vi "Get VIPM Package Installed Filepaths.vi"(8 "error in (no error)":errorcluster, 9 "LabVIEW version in":string, 11 "spec INI refnum in":T1) -> (0 "error out":errorcluster, 1 "LabVIEW version out":string, 2 "Installed Filepaths":path[](array[path]), 3 "spec INI refnum out":T1)   [LabVIEW 2014, in "vipm-to-nipm-package-converter.lvlib"]
doc: "Returns an array of all the installed VIPM package's filepaths for a specific version of LabVIEW.\n\nINPUT(S):\n<b>LabVIEW version</b>: Specifies the LabVIEW version for the NIPM package to support (\"14.0\", \"14.0 (64-bit)\", \"18.0\", \"18.0 (64-bit)\", etc)"
uses:
  vipm-to-nipm-package-converter.lvlib
  <vilib>/Utility/config.llb/Config Data RefNum.ctl
  <vilib>/Utility/sysdir.llb/System Directory Type.ctl
  <vilib>/Utility/config.llb/Read Key (String).vi
  <vilib>/Utility/config.llb/NI_LVConfig.lvlib
panel:
  out "Installed Filepaths (before)":string[](array[string])
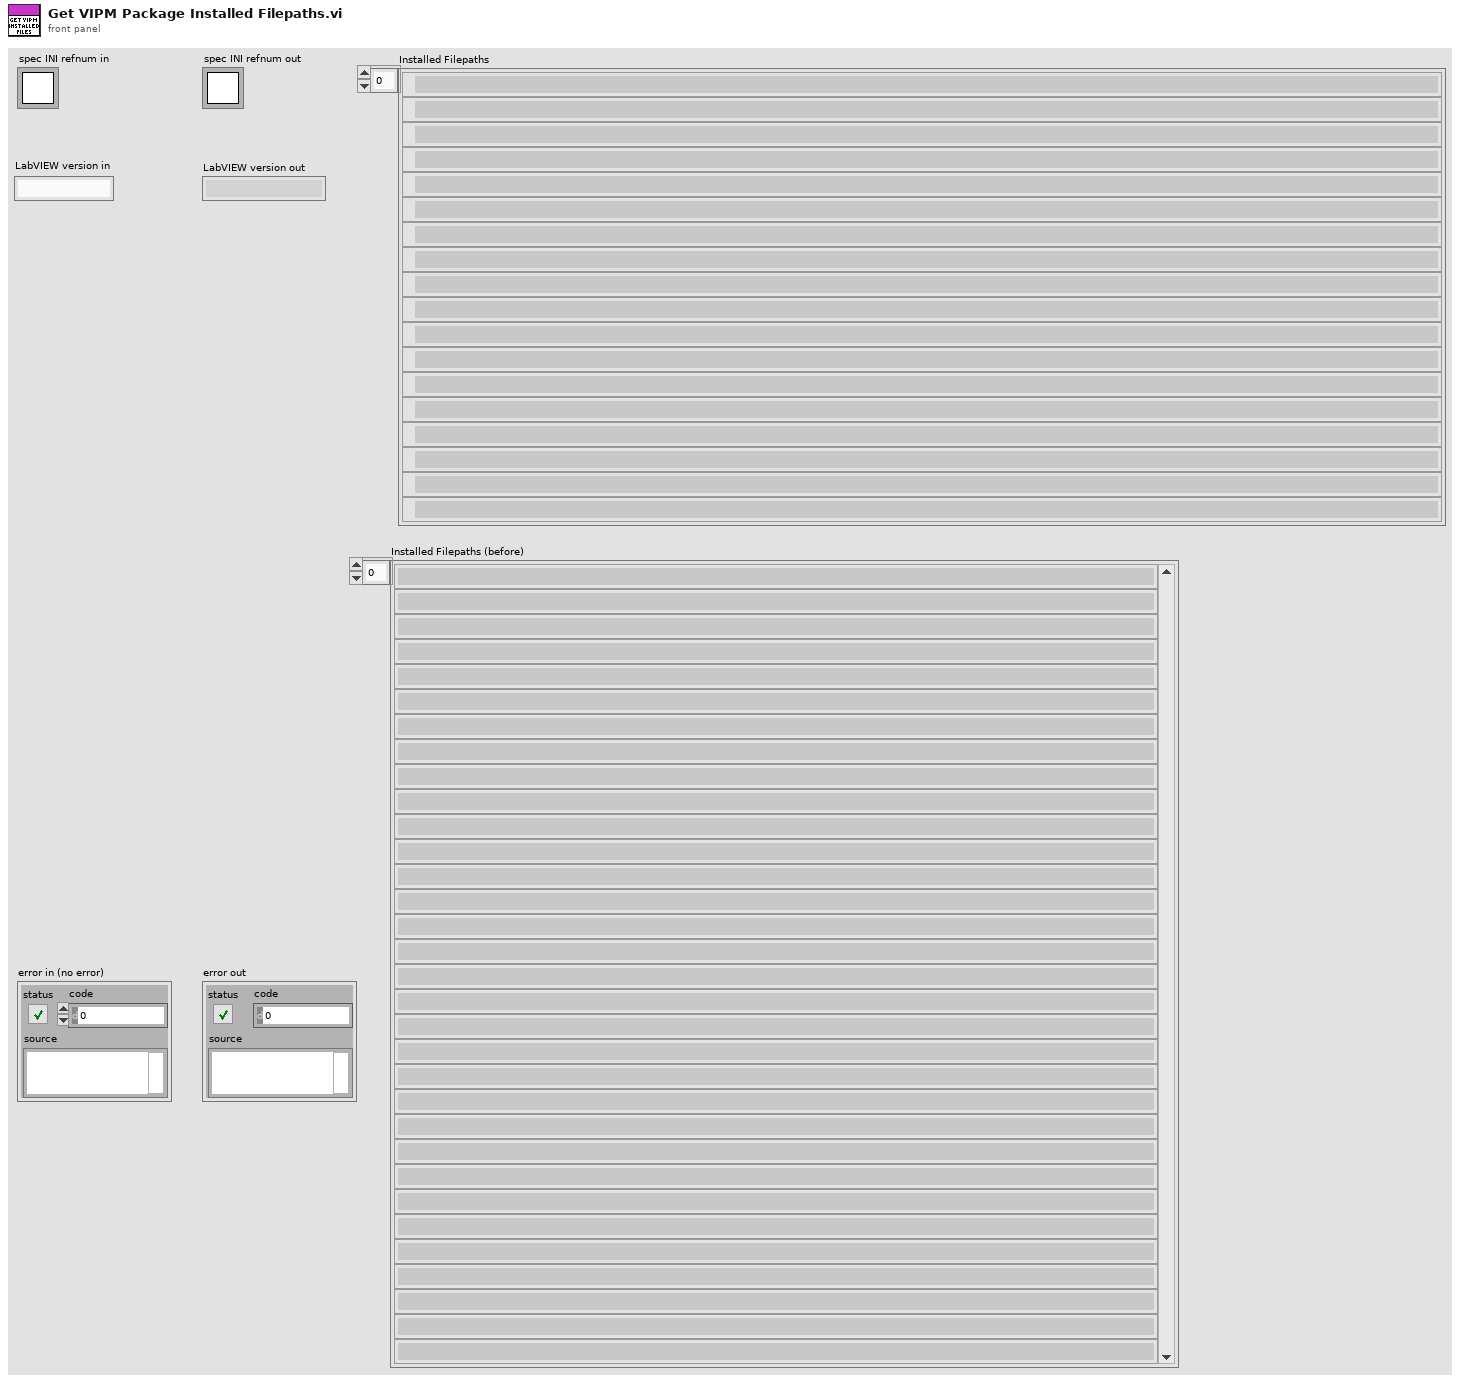
[diagram p1: front panel]
types:
  T1 = typedef "NI_LVConfig.lvlib/Config Data RefNum.ctl" = refnum<k1>
  T2 = typedef "System Directory Type.ctl" = i32
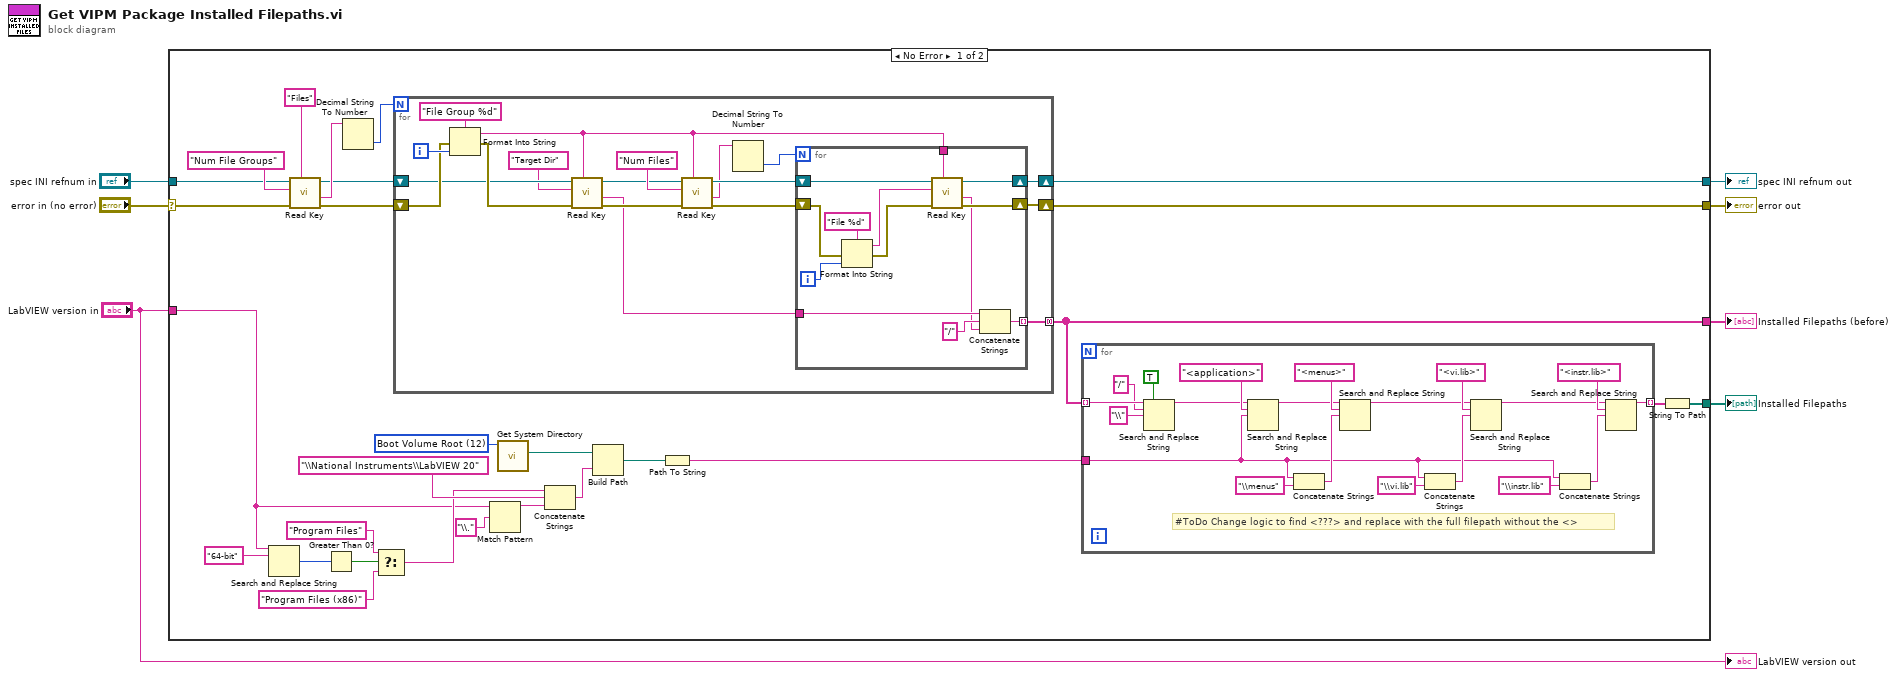
[diagram p0: block diagram]
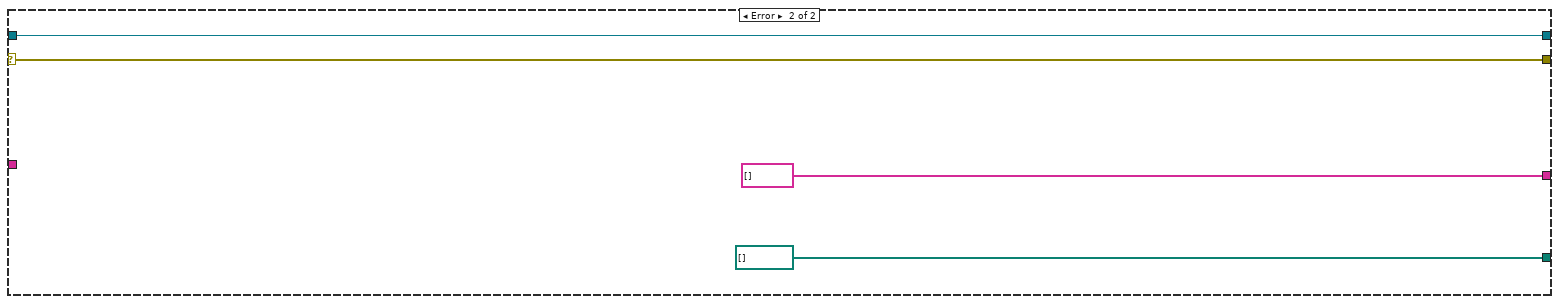
[diagram p2: hidden frame]
diagram:
  n1 = case shown="No Error" "error in (no error)" {
    selector: "error in (no error)" -> [w8 w89]
    tunnel: [w31 w90] -> w7
    tunnel: [w29 w89] -> w6
    tunnel: [w25 string[] []] -> w5
    tunnel: [w19 path[] []] -> w4
    tunnel: "spec INI refnum in" -> [w10 w90]
    tunnel: "LabVIEW version in" -> [w9 _]
    frame No Error {
      w27 = T2 12 items=["User Home"=0, "User Desktop"=1, "User Documents"=2, "User Application Data"=3, "User Preferences"=4, "User Temporary"=5, "Public Documents"=6, "Public Application Data"=7, "Public Preferences"=8, "Public Cache"=13, "System Core Libraries"=9, "System Installed Libraries"=10, "Application Files"=11, "Boot Volume Root"=12] ("system directory type")
      n2 = Search and Replace String(input string=w9, search string="64-bit") -> (number of replacements=w17:i32)  [unwired: 6 in, 3 out]
      n3 = call-poly <vilib>:"Read Key.vi"("section"="Files", "error in (no error)"=w8, "key"="Num File Groups", "refnum"=w10) -> ("error out"=w28:errorcluster, "value"=w34:string, "refnum out"=w30:T1)  [unwired: 4 in, 1 out]
      n4 = Greater Than 0?(x=w17) -> (x > 0?=w16:bool)
      n5 = Decimal String To Number(string=w34) -> (number=w35:i32)  [unwired: 2 in, 1 out]
      n6 = Select(t="Program Files" ("search string"), s=w16, f="Program Files (x86)" ("search string")) -> (s? t:f=w11:string)
      n7 = for {
        N: w35 -> [_]
        shift-right: [w65] -> w29
        shift-left: w28 -> [w72]
        shift-right: [w67] -> w31
        shift-left: w30 -> [w61]
        tunnel: [w56] -> w25 mode=concatenating
        i -> [w73]
        n8 = Format Into String(format string="File Group %d", error in=w72, w73) -> (resulting string=w58:string, error out=w71:errorcluster)  [unwired: 1 in]
        n9 = call-poly <vilib>:"Read Key.vi"("section"=w58, "error in (no error)"=w71, "key"="Target Dir", "refnum"=w61) -> ("error out"=w62:errorcluster, "value"=w57:string, "refnum out"=w60:T1)  [unwired: 4 in, 1 out]
        n10 = call-poly <vilib>:"Read Key.vi"("section"=w58, "error in (no error)"=w62, "key"="Num Files", "refnum"=w60) -> ("error out"=w66:errorcluster, "value"=w64:string, "refnum out"=w68:T1)  [unwired: 4 in, 1 out]
        n11 = Decimal String To Number(string=w64) -> (number=w63:i32)  [unwired: 2 in, 1 out]
        n12 = for {
          N: w63 -> [_]
          shift-right: [w84] -> w67
          shift-left: w68 -> [w85]
          shift-right: [w86] -> w65
          shift-left: w66 -> [w80]
          tunnel: w58 -> [w83]
          tunnel: w57 -> [w78]
          tunnel: [w75] -> w56 mode=indexing
          i -> [w82]
          n13 = Format Into String(format string="File %d", error in=w80, w82) -> (resulting string=w76:string, error out=w79:errorcluster)  [unwired: 1 in]
          n14 = call-poly <vilib>:"Read Key.vi"("section"=w83, "error in (no error)"=w79, "key"=w76, "refnum"=w85) -> ("error out"=w86:errorcluster, "value"=w74:string, "refnum out"=w84:T1)  [unwired: 4 in, 1 out]
          n15 = Concatenate Strings(w78, "/" ("string"), w74) -> (w75:string)
        }
      }
      n16 = Match Pattern(string=w9, regular expression="\\.") -> (before substring=w12:string)  [unwired: 1 in, 3 out]
      n17 = call <vilib>:"Get System Directory.vi"("system directory type"=w27) -> ("system directory"=w26:path)  [unwired: 10 in]
      n18 = Concatenate Strings(w11, "\\National Instruments\\LabVIEW 20" ("name or relative path"), w12) -> (w23:string)
      n19 = Build Path(base path=w26, name or relative path=w23) -> (appended path=w22:path)
      n20 = Path To String(path=w22) -> (string=w21:string)
      n21 = for {
        tunnel: w25 -> [w54] mode=indexing
        tunnel: w21 -> [w36]
        tunnel: [w37] -> w20 mode=indexing
        # "#ToDo Change logic to find <???> and replace with the full filepath without the <>"
        n22 = Search and Replace String(replace all?=TRUE ("replace all? (F)"), input string=w54, search string="/", replace string="\\" ("replace string (\"\")")) -> (result string=w53:string)  [unwired: 4 in, 3 out]
        n23 = Search and Replace String(input string=w53, search string="<application>", replace string=w36) -> (result string=w46:string)  [unwired: 5 in, 3 out]
        n24 = Concatenate Strings(w36, "\\menus" ("string")) -> (w47:string)
        n25 = Search and Replace String(input string=w46, search string="<menus>", replace string=w47) -> (result string=w42:string)  [unwired: 5 in, 3 out]
        n26 = Concatenate Strings(w36, "\\vi.lib" ("string")) -> (w45:string)
        n27 = Search and Replace String(input string=w42, search string="<vi.lib>", replace string=w45) -> (result string=w38:string)  [unwired: 5 in, 3 out]
        n28 = Concatenate Strings(w36, "\\instr.lib" ("string")) -> (w39:string)
        n29 = Search and Replace String(input string=w38, search string="<instr.lib>", replace string=w39) -> (result string=w37:string)  [unwired: 5 in, 3 out]
      }
      n30 = String To Path(string=w20) -> (path=w19:path[])
    }
    frame Error {
    }
  }
  "Installed Filepaths (before)" <- w5
  "spec INI refnum out" <- w7
  "error out" <- w6
  "Installed Filepaths" <- w4
  "LabVIEW version out" <- "LabVIEW version in"
